vi "EtherCAT Mini-DAQ VI.vi"() -> ()   [LabVIEW 2019]
panel:
  in  "Path":path=path "C:/DAQ.lvm"
  in  "Test Runtime (s)":dbl=60.0
  in  "Sample Rate (Hz)":dbl=32.0
  out "Euler X":dbl(graph)
  out "Euler Y":dbl(graph)
  out "Euler Z":dbl(graph)
  out "Analogue Channel 2":dbl(graph)
  in  "Stop":bool
  out "Analogue Channel 1":dbl(graph)
  out "Analogue Channel 7":dbl(graph)
  out "Analogue Channel 6":dbl(graph)
  out "Analogue Channel 5":dbl(graph)
  out "Analogue Channel 4":dbl(graph)
  out "Analogue Channel 3":dbl(graph)
  out "Analogue Channel 8":dbl(graph)
  # "EtherCAT Mini-DAQ Data Aquisition System"
  # "Analogue Channels"
  # "Digital IMU Channels"
  # "16-bit resolution, reccomended sampling frequency 32Hz"
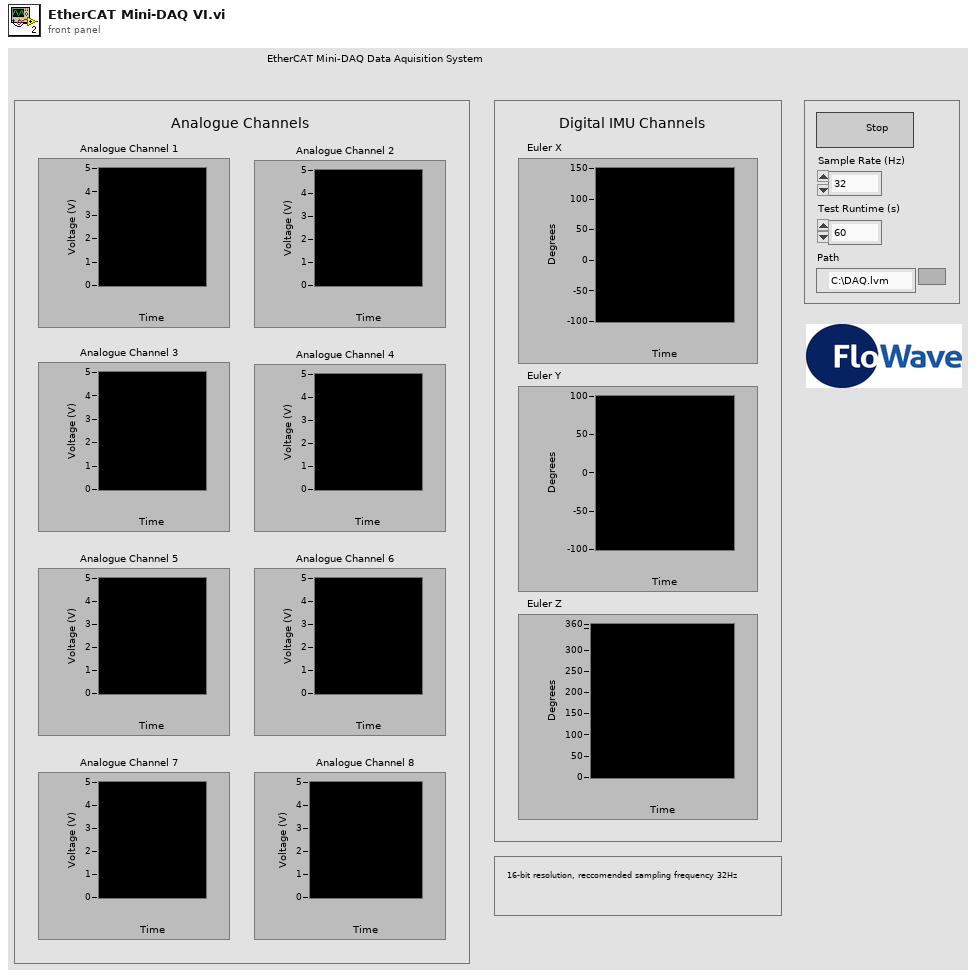
[diagram p1: front panel]
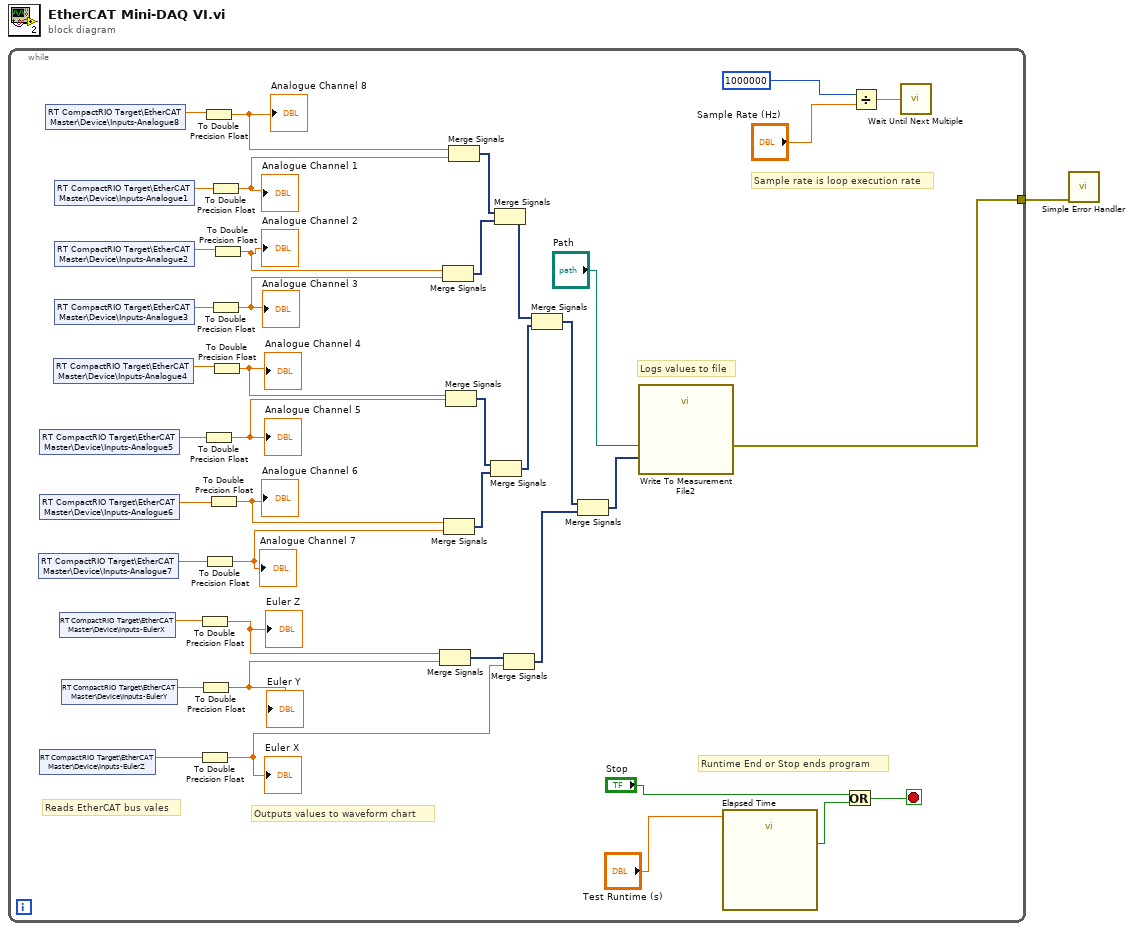
[diagram p0: block diagram]
diagram:
  n1 = while {
    tunnel: [w40] -> w1
    stop <- w2 stop-if-true
    # "Logs values to file"
    # "Outputs values to waveform chart"
    # "Reads EtherCAT bus vales"
    # "Sample rate is loop execution rate"
    # "Runtime End or Stop ends program"
    n2 = shared-variable "RT CompactRIO Target\\EtherCAT Master\\Device\\Inputs-Analogue7"() -> (w34:sgl)  [unwired: 1 in, 1 out]
    n3 = shared-variable "RT CompactRIO Target\\EtherCAT Master\\Device\\Inputs-Analogue5"() -> (w36:sgl)  [unwired: 1 in, 1 out]
    n4 = shared-variable "RT CompactRIO Target\\EtherCAT Master\\Device\\Inputs-Analogue6"() -> (w35:sgl)  [unwired: 1 in, 1 out]
    n5 = shared-variable "RT CompactRIO Target\\EtherCAT Master\\Device\\Inputs-EulerZ"() -> (w23:sgl)  [unwired: 1 in, 1 out]
    n6 = shared-variable "RT CompactRIO Target\\EtherCAT Master\\Device\\Inputs-Analogue8"() -> (w42:sgl)  [unwired: 1 in, 1 out]
    n7 = shared-variable "RT CompactRIO Target\\EtherCAT Master\\Device\\Inputs-Analogue4"() -> (w37:sgl)  [unwired: 1 in, 1 out]
    n8 = shared-variable "RT CompactRIO Target\\EtherCAT Master\\Device\\Inputs-Analogue1"() -> (w41:sgl)  [unwired: 1 in, 1 out]
    n9 = shared-variable "RT CompactRIO Target\\EtherCAT Master\\Device\\Inputs-Analogue2"() -> (w39:sgl)  [unwired: 1 in, 1 out]
    n10 = shared-variable "RT CompactRIO Target\\EtherCAT Master\\Device\\Inputs-Analogue3"() -> (w38:sgl)  [unwired: 1 in, 1 out]
    n11 = shared-variable "RT CompactRIO Target\\EtherCAT Master\\Device\\Inputs-EulerX"() -> (w25:sgl)  [unwired: 1 in, 1 out]
    n12 = shared-variable "RT CompactRIO Target\\EtherCAT Master\\Device\\Inputs-EulerY"() -> (w24:sgl)  [unwired: 1 in, 1 out]
    n13 = To Double Precision Float(number=w25) -> (double precision float=w22:dbl)
    "Euler Z" <- w22
    n14 = To Double Precision Float(number=w23) -> (double precision float=w7:dbl)
    "Euler X" <- w7
    n15 = To Double Precision Float(number=w24) -> (double precision float=w21:dbl)
    "Euler Y" <- w21
    n16 = To Double Precision Float(number=w42) -> (double precision float=w33:dbl)
    "Analogue Channel 8" <- w33
    n17 = To Double Precision Float(number=w36) -> (double precision float=w30:dbl)
    "Analogue Channel 5" <- w30
    n18 = To Double Precision Float(number=w34) -> (double precision float=w28:dbl)
    "Analogue Channel 7" <- w28
    n19 = To Double Precision Float(number=w35) -> (double precision float=w29:dbl)
    "Analogue Channel 6" <- w29
    n20 = To Double Precision Float(number=w41) -> (double precision float=w27:dbl)
    "Analogue Channel 1" <- w27
    n21 = To Double Precision Float(number=w38) -> (double precision float=w32:dbl)
    "Analogue Channel 3" <- w32
    n22 = To Double Precision Float(number=w37) -> (double precision float=w31:dbl)
    "Analogue Channel 4" <- w31
    n23 = To Double Precision Float(number=w39) -> (double precision float=w26:dbl)
    "Analogue Channel 2" <- w26
    n24 = Merge Signals(w22, w21) -> (w20:dynamicdata)
    n25 = Merge Signals(w26, w32) -> (w16:dynamicdata)
    n26 = Merge Signals(w29, w28) -> (w19:dynamicdata)
    n27 = Merge Signals(w31, w30) -> (w18:dynamicdata)
    n28 = Merge Signals(w33, w27) -> (w17:dynamicdata)
    n29 = Merge Signals(w18, w19) -> (w15:dynamicdata)
    n30 = Merge Signals(w17, w16) -> (w14:dynamicdata)
    n31 = Merge Signals(w20, w7) -> (w13:dynamicdata)
    n32 = Merge Signals(w14, w15) -> (w12:dynamicdata)
    n33 = Merge Signals(w12, w13) -> (w11:dynamicdata)
    n34 = call "Write To Measurement File2"("Signals"=w11, "Filename"="Path") -> ("error out"=w40:errorcluster)  [unwired: 15 in, 2 out]
    n35 = call "Elapsed Time"("Time Target (s)"="Test Runtime (s)") -> ("Time has Elapsed"=w3:bool)  [unwired: 11 in, 7 out]
    n36 = Or(x="Stop", y=w3) -> (x .or. y?=w2:bool)
    n37 = Divide(x=u32 1000000 ("Tick Count(uSec)"), y="Sample Rate (Hz)") -> (x/y=w8:dbl)
    n38 = call "Wait Until Next Multiple"("Count(uSec)"=w8) -> ()  [unwired: 1 out]
  }
  n39 = call <vilib>:"Simple Error Handler.vi"("error in (no error)"=w1) -> ()  [unwired: 1 in, 8 out]
